vi "U_BendTwist_2_U_z.vi"(9 "AO offset [V]":fxp<+,25,3>=2.3499999046325684, 10 "U_twist [V]":fxp<+/-,26,4>, 11 "U_Bend [V]":fxp<+/-,26,4>) -> (2 "AO_coil3 [V]":fxp<+,25,3>, 3 "AO_coil2 [V]":fxp<+,25,3>)   [LabVIEW 2017, in "FPGA functions.lvlib"]
doc: "Convert bend and twist control efforts into z-direction control efforts"
uses:
  FPGA functions.lvlib
  <vilib>/Platform/TimedLoop/XDataNode/XDataNode.xnode
  <vilib>/Platform/TimedLoop/XDataNode/nitl_modes.ctl
  <vilib>/Platform/TimedLoop/XDataNode/XDNodeRunTimeDep.lvlib
  <vilib>/Platform/TimedLoop/XDataNode/wakeup.ctl
  <vilib>/Platform/TimedLoop/XDataNode/timing_clust.ctl
  <vilib>/rvi/FXPMathLib/FxpAdd/XNode/nifxpmath_Add.xnode
  <vilib>/rvi/FXPMathLib/sim/FxpSim.dll
  <vilib>/rvi/FXPMathLib/FxpSub/XNode/nifxpmath_Sub.xnode
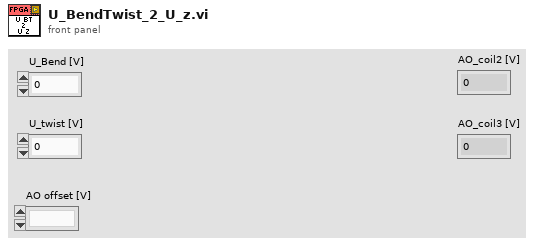
[diagram p1: front panel]
types:
  T1 = typedef "XDNodeRunTimeDep.lvlib/timing_clust.ctl" = cluster{"Expected End [f-1]":u64, "Actual End [f-1]":u64, "Finished Late? [f-1]":bool, "Expected End [i-1]":u64, "Actual End [i-1]":u64, "Finished Late? [i-1]":bool, "Expected Start [i]":u64, "Actual Start [i]":u64, "Expected Start [f]":u64, "Actual Start [f]":u64, "Source Name":string, "Structure Name":string, "Period":i64, "Deadline":i64, "Offset":i64, "Start":i64, "Priority":i32, "Timeout":i32, "Mode":T2, "Wakeup Reason":T3, "Error":errorcluster, "Source Type":string, "Secondary Source Type":string, "Global End Time":u64, "Global Start Time":u64, "Frame Duration":u64, "Iteration Duration":u64, "Assigned CPU":i32, "I/O Scan Engine Mode":u32}
  T2 = typedef "XDNodeRunTimeDep.lvlib/nitl_modes.ctl" = enum32{"No Change", "Process missed periods, maintain original phase", "Discard missed periods, maintain original phase", "Process missed periods, ignore original phase", "Discard missed periods, ignore original phase"}
  T3 = typedef "XDNodeRunTimeDep.lvlib/wakeup.ctl" = enum32{"Normal", "Aborted", "Asynchronous wakeup", "Timing source error", "Timed loop error", "Timeout"}
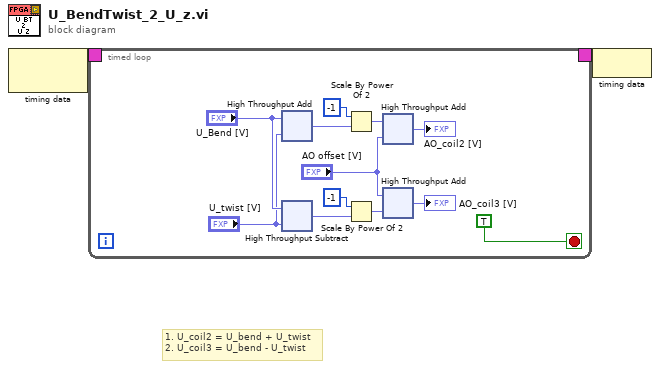
[diagram p0: block diagram]
diagram:
  # "1. U_coil2 = U_bend + U_twist\n2. U_coil3 = U_bend - U_twist"
  n1 = node-c288() -> (w2:T1)  [unwired: 1 in]
  n2 = timed-loop {
    timing: w2 -> [_]
    timing-out: [_] -> w1
    stop <- TRUE stop-if-true
    n3 = xnode ("High Throughput Add")("x"="U_Bend [V]", "y"="U_twist [V]") -> ("x+y"=w4:fxp<+/-,28,5>)
    n4 = xnode ("High Throughput Subtract")("x"="U_Bend [V]", "y"="U_twist [V]") -> ("x-y"=w5:fxp<+/-,28,5>)
    n5 = Scale By Power Of 2(n=i16 -1, x=w4) -> (x*2^n=w3:fxp<+/-,28,5>)
    n6 = Scale By Power Of 2(n=i16 -1, x=w5) -> (x*2^n=w6:fxp<+/-,28,5>)
    n7 = xnode ("High Throughput Add")("x"=w3, "y"="AO offset [V]") -> ("x+y"=→"AO_coil2 [V]":fxp<+,25,3>)
    n8 = xnode ("High Throughput Add")("x"="AO offset [V]", "y"=w6) -> ("x+y"=→"AO_coil3 [V]":fxp<+,25,3>)
  }
  n9 = node-c288(w1) -> ()
